vi "Configure Bus Source (AUDIO - Data).vi"(0 "VISA resource name":refnum<visa-resource-name>, 1 "Data Size (8)":i32=8, 5 "BUS Number (9: Bus 1)":u16(ring)=9 items=["Bus 1"=9, "Bus 2"=10, "Bus 3"=11, "Bus 4"=12], 7 "Data Source (0: Channel 1)":u16(ring) items=["Channel 1"=0, "Channel 2"=1, "Channel 3"=2, "Channel 4"=3, "Digital Channel 0"=14, "Digital Channel 1"=15, "Digital Channel 2"=16, "Digital Channel 3"=17, "Digital Channel 4"=18, "Digital Channel 5"=19, "Digital Channel 6"=20, "Digital Channel 7"=21, "Digital Channel 8"=22, "Digital Channel 9"=23, "Digital Channel 10"=24, "Digital Channel 11"=25, "Digital Channel 12"=26, "Digital Channel 13"=27, "Digital Channel 14"=28, "Digital Channel 15"=29], 9 "Data Polarity (0: Normal)":u16(ring) items=["Normal", "Invert"], 11 "error in (no error)":errorcluster) -> (4 "VISA resource name out":refnum<visa-resource-name>, 15 "error out":errorcluster)   [LabVIEW 2010, in "Tektronix DPO MSO 2000 4000 Series.lvlib"]
doc: "This VI configures the data settings for the AUDIO bus.\n\n<B>Note:</B> This VI is only valid if you have installed the AUDIO application module."
uses:
  <instrlib>/Tektronix DPO MSO 2000 4000 Series/Tektronix DPO MSO 2000 4000 Series.lvlib
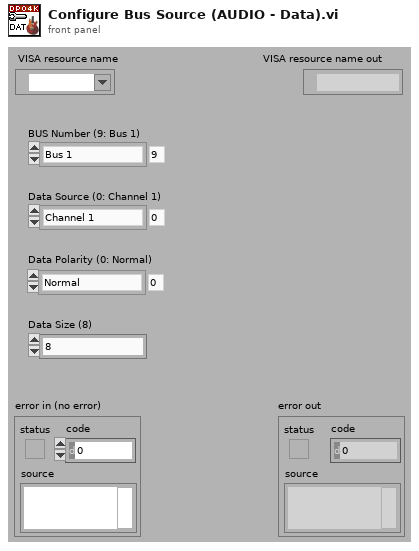
[diagram p1: front panel]
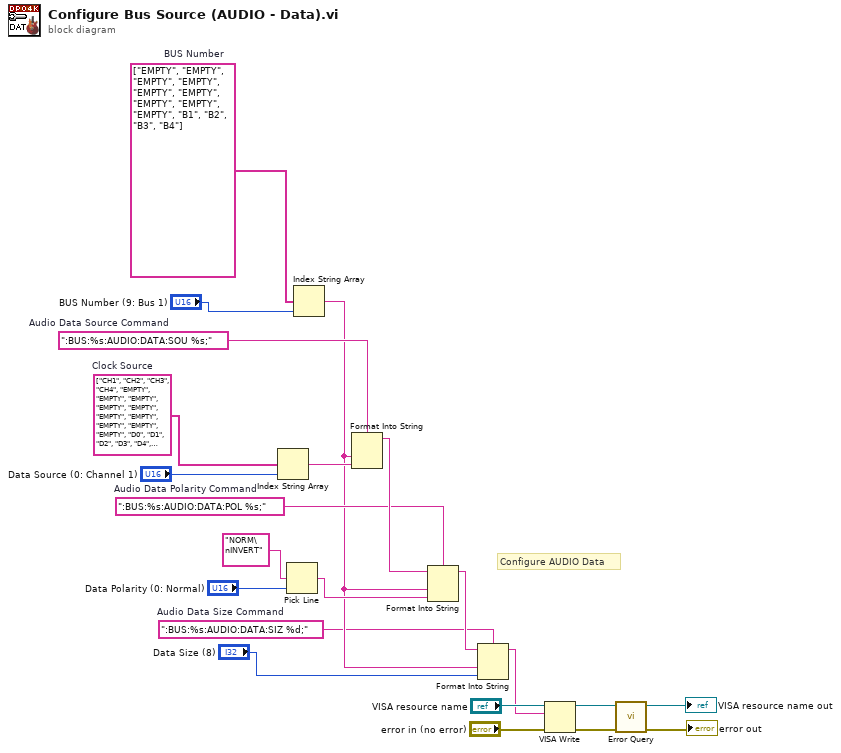
[diagram p0: block diagram]
diagram:
  w8 = ":BUS:%s:AUDIO:DATA:SIZ %d;"  # Audio Data Size Command
  w12 = ":BUS:%s:AUDIO:DATA:POL %s;"  # Audio Data Polarity Command
  w20 = string[] ["CH1", "CH2", "CH3", "CH4", "EMPTY", "EMPTY", "EMPTY", "EMPTY", "EMPTY", "EMPTY", "EMPTY", "EMPTY", "EMPTY", "EMPTY", "D0", "D1", "D2", "D3", "D4", "D5", "D6", "D7", "D8", "D9", "D10", "D11", "D12", "D13", "D14", "D15"]  # Clock Source
  w21 = ":BUS:%s:AUDIO:DATA:SOU %s;"  # Audio Data Source Command
  w22 = string[] ["EMPTY", "EMPTY", "EMPTY", "EMPTY", "EMPTY", "EMPTY", "EMPTY", "EMPTY", "EMPTY", "B1", "B2", "B3", "B4"]  # BUS Number
  # "Configure AUDIO Data"
  n1 = Index String Array(1:"Data Source (0: Channel 1)", 2:w20) -> (0:w18:string)  [unwired: 1 in]
  n2 = Pick Line(multi-line string="NORM\nINVERT", line index="Data Polarity (0: Normal)") -> (output string=w14:string)  [unwired: 1 in]
  n3 = Index String Array(1:"BUS Number (9: Bus 1)", 2:w22) -> (0:w10:string)  [unwired: 1 in]
  n4 = Format Into String(format string=w21, w10, w18) -> (resulting string=w13:string)  [unwired: 2 in, 1 out]
  n5 = Format Into String(format string=w12, initial string=w13, w10, w14) -> (resulting string=w11:string)  [unwired: 1 in, 1 out]
  n6 = Format Into String(format string=w8, initial string=w11, w10, "Data Size (8)") -> (resulting string=w6:string)  [unwired: 1 in, 1 out]
  n7 = VISA Write(VISA resource name="VISA resource name", write buffer=w6, error in (no error)="error in (no error)") -> (VISA resource name out=w4:refnum<visa-resource-name>, error out=w3:errorcluster)  [unwired: 1 out]
  n8 = call <instrlib>:"Error Query.vi"("error in (no error)"=w3, "VISA resource name"=w4) -> ("error out"=→"error out":errorcluster, "VISA resource name out"=→"VISA resource name out":refnum<visa-resource-name>)  [unwired: 6 in, 2 out]
